vi "Chart control manipulation.vi"(4 "Visible 3":bool, 6 "Visible 2":bool, 8 "3rd module":dbl, 9 "2nd module":dbl, 10 "1st module":dbl, 11 "Protons position":i32) -> (1 "Energy from module":dbl, 3 "Outside module?":bool)   [LabVIEW 2020]
doc: "Important Vi to control contnent of chart and values of energy \nProton's position is used to check if proton is inside or outside module. (Furthermore, visibility of modules are also included) If not, the speed is constant. If it is inside any module, its energy is computed by combining energy from modules with its previous energy."
panel:
  # "This subvi computes energy from modules"
  # "This instance finds if proton is outside module"
  # "The activation of modules"
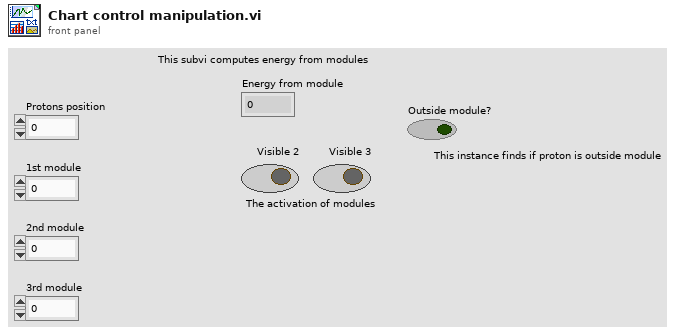
[diagram p1: front panel]
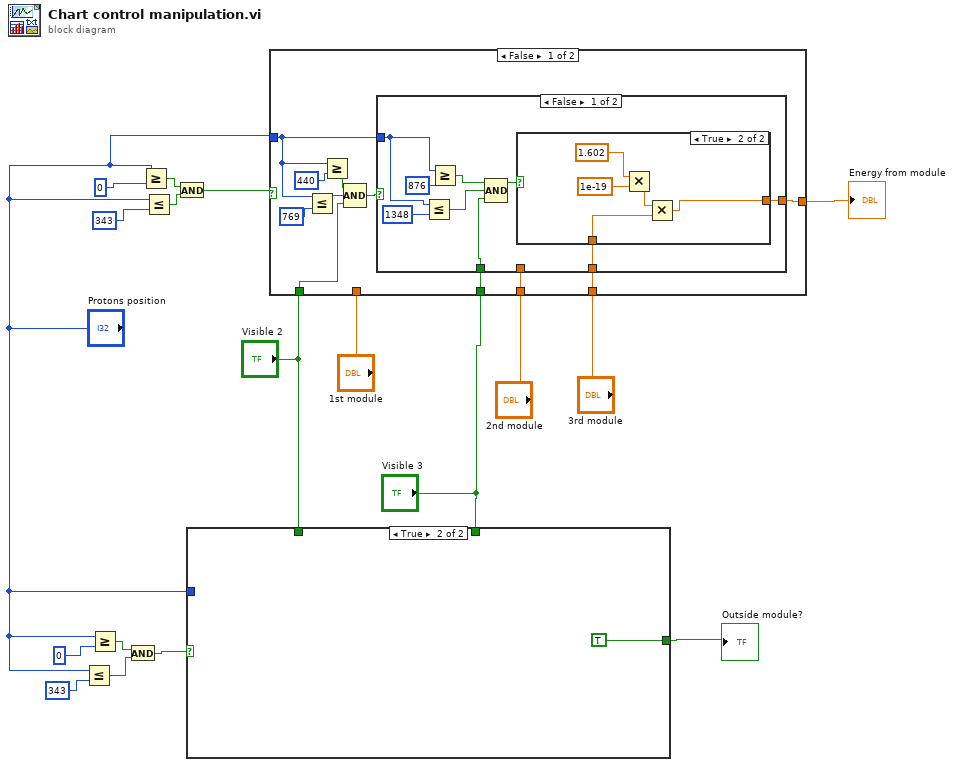
[diagram p0: block diagram]
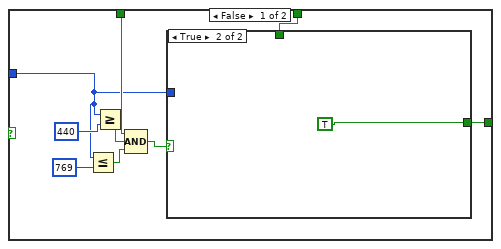
[diagram p2: hidden frame]
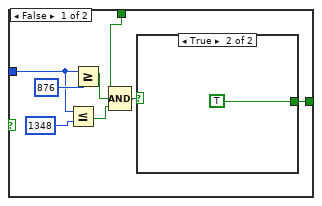
[diagram p3: hidden frame]
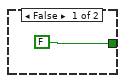
[diagram p4: hidden frame]
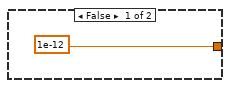
[diagram p5: hidden frame]
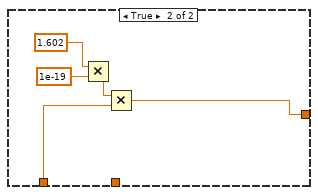
[diagram p6: hidden frame]
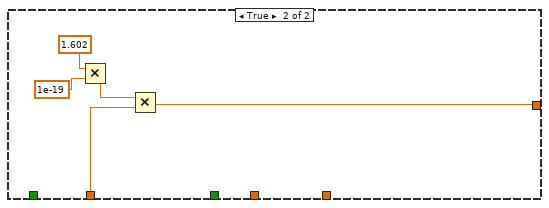
[diagram p7: hidden frame]
diagram:
  n1 = Less Or Equal?(x="Protons position", y=343) -> (x <= y?=w9:bool)
  n2 = Greater Or Equal?(x="Protons position", y=0) -> (x >= y?=w8:bool)
  n3 = And(x=w8, y=w9) -> (x .and. y?=w7:bool)
  n4 = Greater Or Equal?(x="Protons position", y=0) -> (x >= y?=w18:bool)
  n5 = Less Or Equal?(x="Protons position", y=343) -> (x <= y?=w17:bool)
  n6 = And(x=w18, y=w17) -> (x .and. y?=w16:bool)
  n7 = case shown="True" w7 {
    tunnel: "Protons position" -> [w21 _]
    tunnel: "Visible 2" -> [w22 _]
    tunnel: "Visible 3" -> [w20 _]
    tunnel: [w19 TRUE] -> w3
    frame False {
      n8 = Less Or Equal?(x=w21, y=769) -> (x <= y?=w27:bool)
      n9 = Greater Or Equal?(x=w21, y=440) -> (x >= y?=w25:bool)
      n10 = Compound Arithmetic op=AND(w22, w25, w27) -> (w23:bool)
      n11 = case shown="True" w23 {
        tunnel: w21 -> [w32 _]
        tunnel: w20 -> [w30 _]
        tunnel: [w28 TRUE] -> w19
        frame False {
          n12 = Less Or Equal?(x=w32, y=1348) -> (x <= y?=w34:bool)
          n13 = Greater Or Equal?(x=w32, y=876) -> (x >= y?=w33:bool)
          n14 = Compound Arithmetic op=AND(w30, w33, w34) -> (w29:bool)
          n15 = case shown="True" w29 {
            tunnel: [FALSE TRUE] -> w28
            frame False {
            }
            frame True {
            }
          }
        }
        frame True {
        }
      }
    }
    frame True {
    }
  }
  "Outside module?" <- w3
  n16 = case shown="False" w16 {
    tunnel: "1st module" -> [_ w72]
    tunnel: [w44 w71] -> w14
    tunnel: "Protons position" -> [w43 _]
    tunnel: "2nd module" -> [w45 _]
    tunnel: "3rd module" -> [w42 _]
    tunnel: "Visible 3" -> [w41 _]
    tunnel: "Visible 2" -> [w40 _]
    frame False {
      n17 = Less Or Equal?(x=w43, y=769) -> (x <= y?=w50:bool)
      n18 = Greater Or Equal?(x=w43, y=440) -> (x >= y?=w48:bool)
      n19 = Compound Arithmetic op=AND(w48, w50, w40) -> (w46:bool)
      n20 = case shown="False" w46 {
        tunnel: w45 -> [_ w67]
        tunnel: [w52 w66] -> w44
        tunnel: w43 -> [w54 _]
        tunnel: w42 -> [w53 _]
        tunnel: w41 -> [w51 _]
        frame False {
          n21 = Less Or Equal?(x=w54, y=1348) -> (x <= y?=w57:bool)
          n22 = Greater Or Equal?(x=w54, y=876) -> (x >= y?=w58:bool)
          n23 = Compound Arithmetic op=AND(w58, w57, w51) -> (w56:bool)
          n24 = case shown="True" w56 {
            tunnel: w53 -> [_ w62]
            tunnel: [1e-12 w61] -> w52
            frame False {
            }
            frame True {
              n25 = Multiply(x=1.602, y=1e-19) -> (x*y=w63:dbl)
              n26 = Multiply(x=w63, y=w62) -> (x*y=w61:dbl)
            }
          }
        }
        frame True {
          n27 = Multiply(x=1.602, y=1e-19) -> (x*y=w68:dbl)
          n28 = Multiply(x=w68, y=w67) -> (x*y=w66:dbl)
        }
      }
    }
    frame True {
      n29 = Multiply(x=1.602, y=1e-19) -> (x*y=w73:dbl)
      n30 = Multiply(x=w73, y=w72) -> (x*y=w71:dbl)
    }
  }
  "Energy from module" <- w14
